vi "GRIMMcontrollerVI.vi"(8 "error in (no error)":errorcluster) -> (0 "error out":errorcluster)   [LabVIEW 2013]
doc: "Use this template to build a VI to use as a subVI."
uses:
  GRIMMstatusEnum.ctl
  GRIMMmeasurementEnum.ctl
  GRIMMErrorMessage.ctl
  GRIMMmeasurementCluster.ctl
  <vilib>/Instr/_visa.llb/VISA Configure Serial Port (Instr).vi
panel:
  in  "Save GRIMM file":bool
  in  "GRIMM File Path":path
  in  "error in (no error) 3":errorcluster
  out "XY Graph 2":cluster{dbl[], dbl[]}[](graph)
  out "Counts vs Time":waveform(dbl)[](graph)
  out "XY Graph":cluster{dbl[], dbl[]}[](graph)
  out "Error Messages":u16(ring) items=["New SELF-TEST: Fault Self-Test"=128, "No Memory Card"=64, "Check Nozzle: Whirls > 5%"=32, "No Operation: Battery Capacity = 0%"=16, "Please Recharge: Battery Capacity < 10%"=8, "Pump Current too High - Motor Current Imot > 100%"=4, "Flow-Error: Volume flow control out of control range"=3, "Check Filter Imot < 20% "=2, "Check Filter Imot > 60%"=1, "No Error :)"=0]
  out "Battery Power (%)":i32
  out "Power Supply Type":T1(ring)
  out "Pump Current (%)":i32
  out "Number of Particles":i32[](array[numeric])
  in  "error in (no error) 2":errorcluster
  in  "Set Interval Time Button":bool
  in  "Interval Time":T2(ring)
  out "read buffer":string
  in  "Stop GRIMM Measurement":bool
  in  "Start GRIMM Measurement":bool
  in  "stop":bool
  in  "GRIMM Com Port":refnum<visa-resource-name>="COM16"
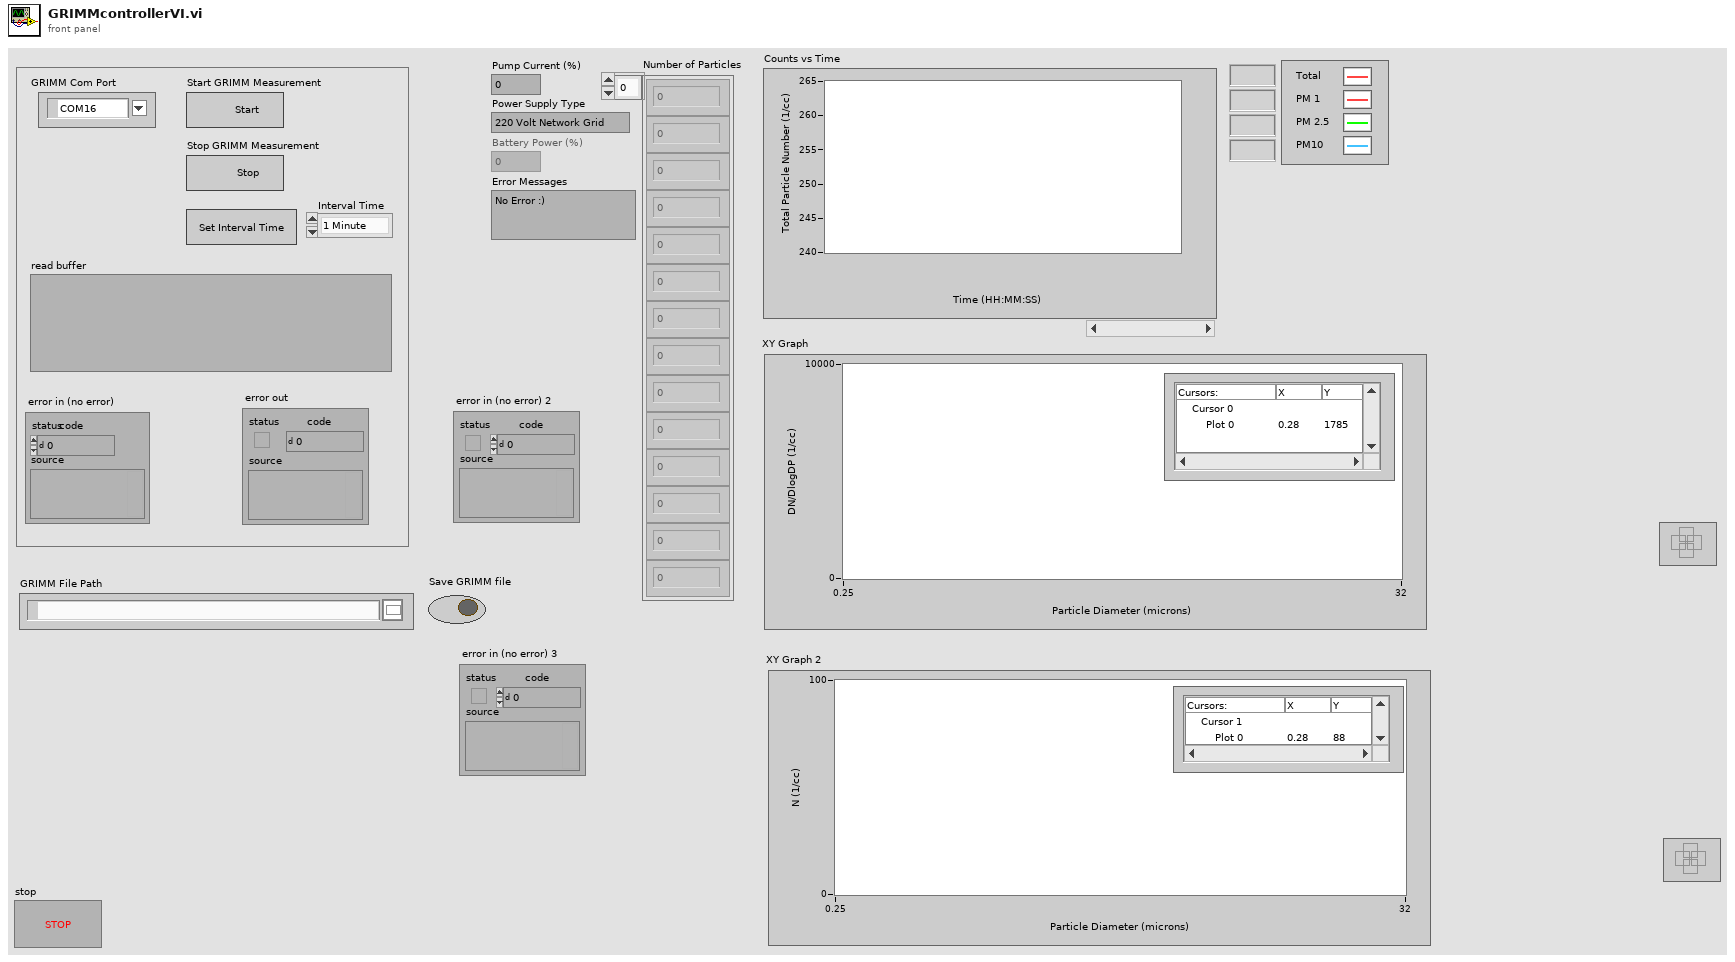
[diagram p1: front panel]
types:
  T1 = enum16{"220 Volt Network Grid", "Battery Powered"}
  T2 = enum16{"1 Minute", "5 Mintues", "10 Minutes", "15 Minutes", "30 Minutes", "60 Minutes", "6 Seconds", "3 Seconds", "2 Seconds", "1 Second"}
  T3 = typedef "GRIMMmeasurementEnum.ctl" = enum16{"Save Raw to file", "Get NvsDiameter", "Get DNDlogDPVsDiameter", "Get CountsVsTime", "Get Raw Data", "InsertMeasurement", "Init"}
  T4 = typedef "GRIMMstatusEnum.ctl" = enum16{"Get Pump Current", "Get Power Supply Type", "Get Battery Power", "Get Error message", "Get Instrument DateTime", "Insert Status Data", "Init"}
  T5 = typedef "GRIMMmeasurementCluster.ctl" = cluster{"Threshold Bin size":dbl[], "Measurement Data":i32[]}
  T6 = enum8{"Enabled", "Disabled", "Disabled and Grayed Out"}
  T7 = typedef "GRIMMErrorMessage.ctl" = u16
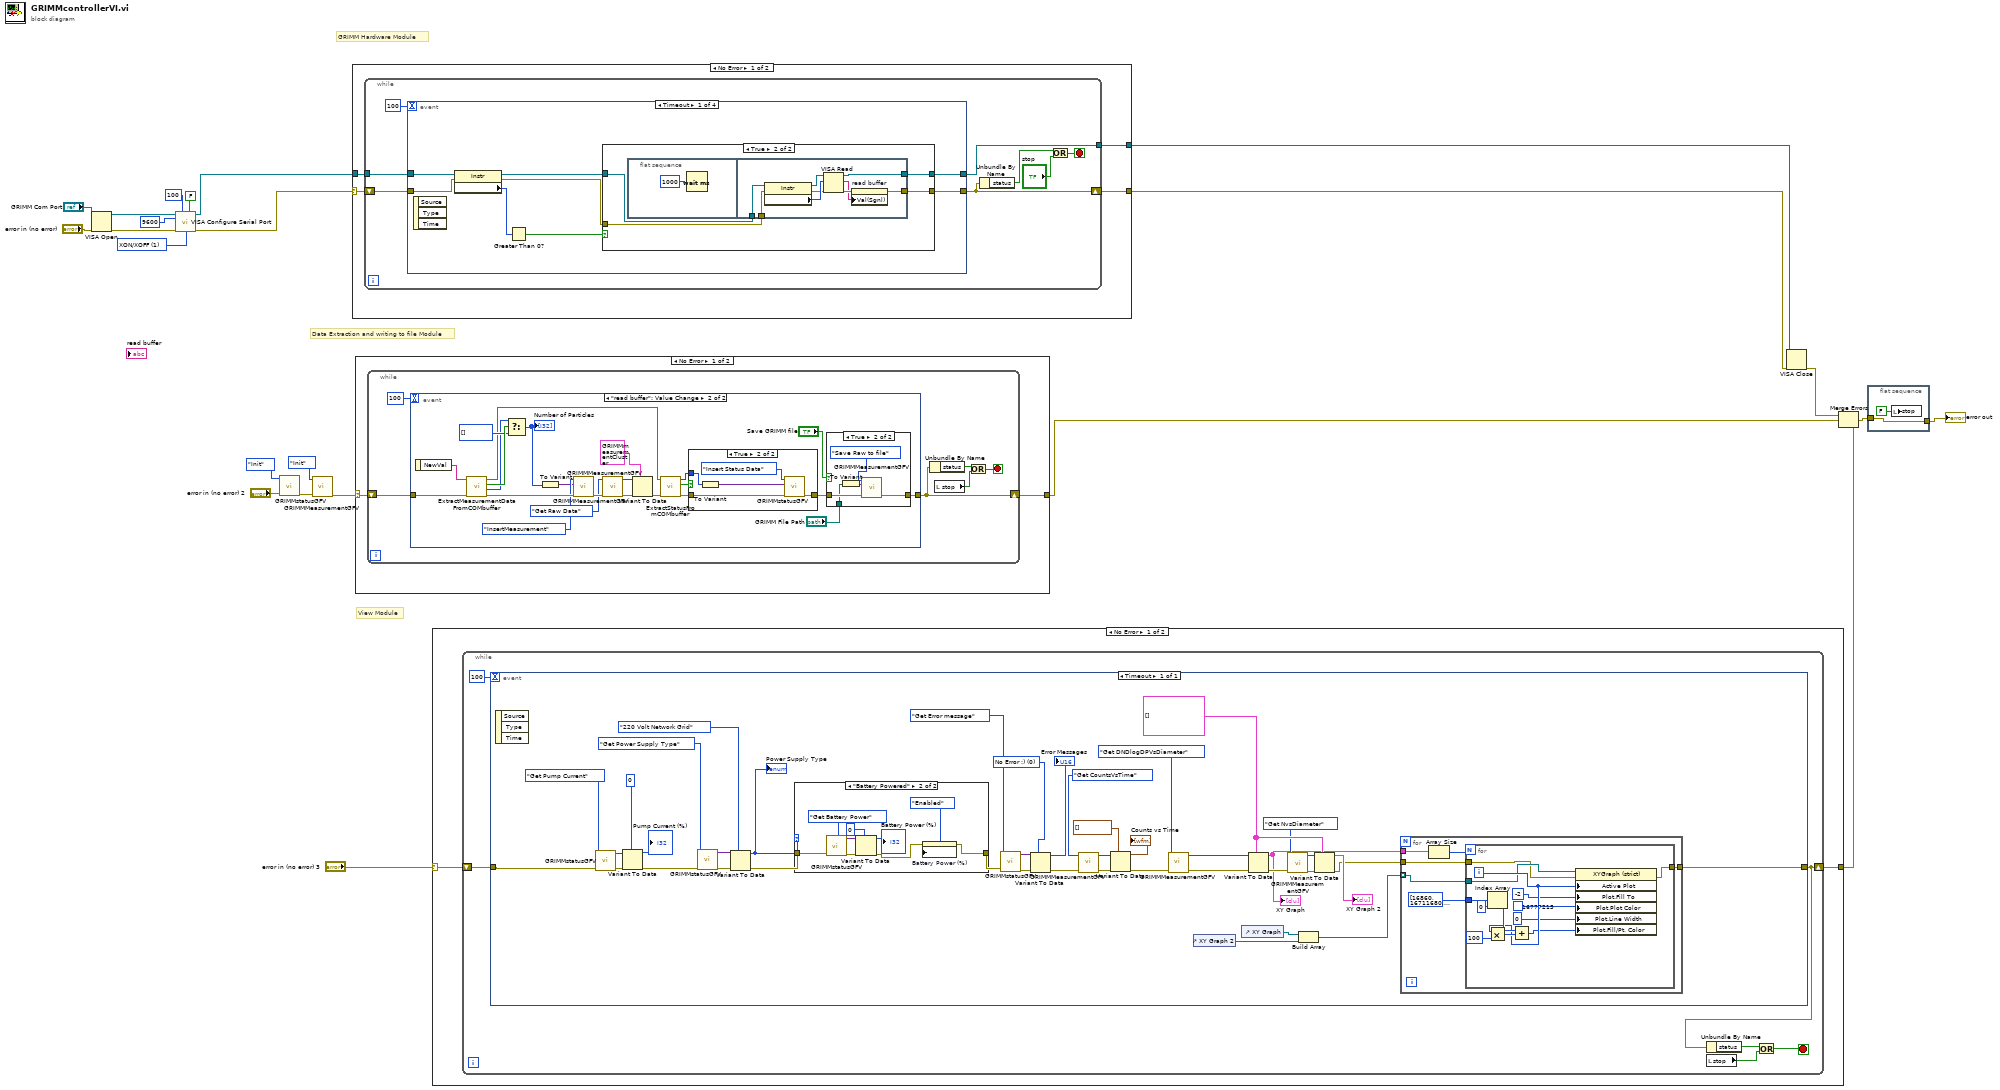
[diagram p0: block diagram]
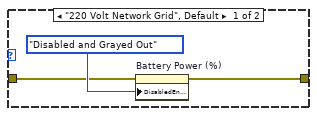
[diagram p2: hidden frame]
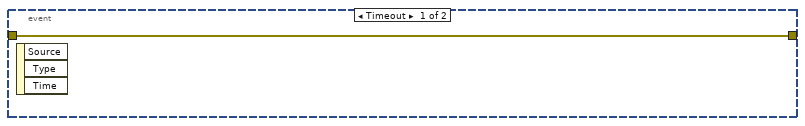
[diagram p4: hidden frame]
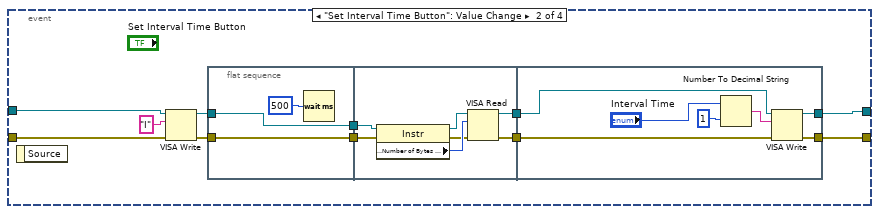
[diagram p9: hidden frame]
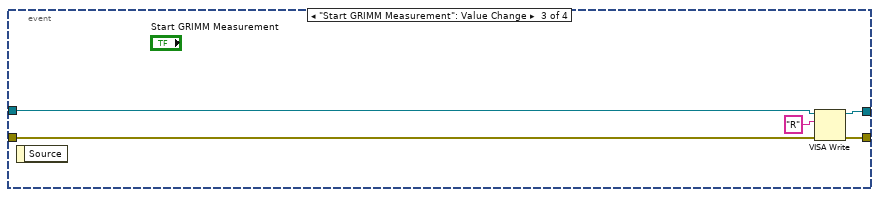
[diagram p10: hidden frame]
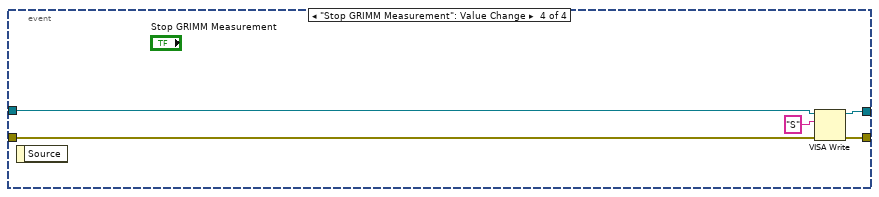
[diagram p11: hidden frame]
diagram:
  w16 = u16 1 items=["None", "XON/XOFF", "RTS/CTS", "XON/XOFF & RTS/CTS", "DTR/DSR", "XON/XOFF & DTR/DSR"] ("flow control (0:none)")
  # "View Module"
  # "Data Extraction and writing to file Module"
  # "GRIMM Hardware Module"
  n1 = VISA Open(error in (no error)="error in (no error)", VISA resource name="GRIMM Com Port") -> (VISA resource name=w23:refnum<visa-resource-name>, error out=w22:errorcluster)  [unwired: 3 in]
  n2 = call-poly "VISA Configure Serial Port"("VISA resource name"=w23, "timeout (10sec)"=u32 100, "Enable Termination\nChar (T)"=FALSE ("Enable Termination\nChar (T)"), "baud rate (9600)"=u32 9600, "error in (no error)"=w22, "flow control (0:none)"=w16) -> ("VISA resource name out"=w13:refnum<visa-resource-name>, "error out"=w15:errorcluster)  [unwired: 8 in]
  n3 = call "GRIMMstatusGFV.vi"("error in (no error)"="error in (no error) 2", "GrimmStatusEnum"=GRIMMstatusEnum."Init") -> ("error out"=w5:errorcluster)  [unwired: 8 in, 1 out]
  n4 = call "GRIMMMeasurementGFV.vi"("error in (no error)"=w5, "GRIMMMeasEnum"=GRIMMmeasurementEnum."Init") -> ("error out"=w3:errorcluster)  [unwired: 8 in, 1 out]
  n5 = case shown="No Error" w15 {
    selector: w15 -> [w26 w99]
    tunnel: [w25 w99] -> w14
    tunnel: w13 -> [w27 w98]
    tunnel: [w24 w98] -> w12
    frame No Error {
      n6 = while {
        tunnel: w27 -> [w34]
        tunnel: [w33] -> w24
        shift-right: [w32] -> w25
        shift-left: w26 -> [w35]
        stop <- w29 stop-if-true
        n7 = event shown="[0] Timeout" {
          selector: _ -> [_ _ _ _]
          dyn-events: _ -> [_ _ _ _]
          timeout: 100 -> [_ _ _ _]
          tunnel: w35 -> [w39 w70 w90 w95]
          tunnel: [w36 w62 w89 w94] -> w32
          tunnel: [w37 w61 w88 w93] -> w33
          tunnel: w34 -> [w43 w69 w91 w96]
          event Timeout {
            n8 = event-data() -> ()  [unwired: 1 in, 3 out]
            n9 = property class="Instr"(reference=w43, error in=w39) -> (reference out=w40:refnum<visa-resource-name>, error out=w38:errorcluster, "Serial Settings:Number of Bytes at Serial Port"=w41:u32)
            n10 = Greater Than 0?(x=w41) -> (x > 0?=w42:bool)
            n11 = case shown="True" w42 {
              tunnel: w40 -> [w44 w49]
              tunnel: w38 -> [w45 w48]
              tunnel: [w44 w47] -> w37
              tunnel: [w45 w46] -> w36
              frame False {
              }
              frame True {
                n12 = flat-sequence {
                  tunnel: w49 -> [w59]
                  tunnel: w48 -> [w56]
                  tunnel: [w54] -> w47
                  tunnel: [w52] -> w46
                  frame #0 {
                    n13 = Wait (ms)(milliseconds to wait=u32 1000) -> ()  [unwired: 1 out]
                  }
                  frame #1 {
                    n14 = property class="Instr"(reference=w59, error in=w56) -> (reference out=w58:refnum<visa-resource-name>, error out=w55:errorcluster, "Serial Settings:Number of Bytes at Serial Port"=w57:u32)
                    n15 = VISA Read(VISA resource name=w58, byte count=w57, error in (no error)=w55) -> (VISA resource name out=w54:refnum<visa-resource-name>, read buffer=w51:string, error out=w53:errorcluster)  [unwired: 1 out]
                    n16 = property on="read buffer" class="Str"(error in=w53, "Val(Sgnl)"=w51) -> (error out=w52:errorcluster)  [unwired: 1 in, 1 out]
                  }
                }
              }
            }
          }
          event "Set Interval Time Button": Value Change {
            n17 = event-data() -> ()  [unwired: 1 in, 1 out]
            n18 = VISA Write(VISA resource name=w69, write buffer="I" ("string"), error in (no error)=w70) -> (VISA resource name out=w67:refnum<visa-resource-name>, error out=w66:errorcluster)  [unwired: 1 out]
            n19 = flat-sequence {
              tunnel: w67 -> [w72]
              tunnel: w66 -> [w71]
              tunnel: [w72] -> w65
              tunnel: [w71] -> w60
              tunnel: w65 -> [w77]
              tunnel: [w76] -> w64
              tunnel: [w75] -> w63
              tunnel: w60 -> [w74]
              tunnel: w64 -> [w85]
              tunnel: w63 -> [w84]
              tunnel: [w83] -> w62
              tunnel: [w82] -> w61
              frame #0 {
                n20 = Wait (ms)(milliseconds to wait=u32 500) -> ()  [unwired: 1 out]
              }
              frame #1 {
                n21 = property class="Instr"(reference=w77, error in=w74) -> (reference out=w80:refnum<visa-resource-name>, error out=w78:errorcluster, "Serial Settings:Number of Bytes at Serial Port"=w79:u32)
                n22 = VISA Read(VISA resource name=w80, byte count=w79, error in (no error)=w78) -> (VISA resource name out=w76:refnum<visa-resource-name>, error out=w75:errorcluster)  [unwired: 2 out]
              }
              frame #2 {
                n23 = Number To Decimal String(number="Interval Time", width (-)=i16 1) -> (decimal integer string=w81:string)
                n24 = VISA Write(VISA resource name=w85, write buffer=w81, error in (no error)=w84) -> (VISA resource name out=w82:refnum<visa-resource-name>, error out=w83:errorcluster)  [unwired: 1 out]
              }
            }
          }
          event "Start GRIMM Measurement": Value Change {
            n25 = event-data() -> ()  [unwired: 1 in, 1 out]
            n26 = VISA Write(VISA resource name=w91, write buffer="R", error in (no error)=w90) -> (VISA resource name out=w88:refnum<visa-resource-name>, error out=w89:errorcluster)  [unwired: 1 out]
          }
          event "Stop GRIMM Measurement": Value Change {
            n27 = event-data() -> ()  [unwired: 1 in, 1 out]
            n28 = VISA Write(VISA resource name=w96, write buffer="S", error in (no error)=w95) -> (VISA resource name out=w93:refnum<visa-resource-name>, error out=w94:errorcluster)  [unwired: 1 out]
          }
        }
        n29 = Unbundle By Name(w32) -> ("status"=w31:bool)
        n30 = Or(x=w31, y="stop") -> (x .or. y?=w29:bool)
      }
    }
    frame Error {
    }
  }
  n31 = case shown="No Error" w3 {
    selector: w3 -> [w101 w144]
    tunnel: [w100 w144] -> w11
    frame No Error {
      n32 = while {
        shift-right: [w105] -> w100
        shift-left: w101 -> [w107]
        stop <- w102 stop-if-true
        n33 = event shown="[1] \"read buffer\": Value Change" {
          selector: _ -> [_ _]
          dyn-events: _ -> [_ _]
          timeout: 100 -> [_ _]
          tunnel: w107 -> [w108 w130]
          tunnel: [w108 w111] -> w105
          event Timeout {
            n34 = event-data() -> ()  [unwired: 1 in, 3 out]
          }
          event "read buffer": Value Change {
            n35 = event-data() -> ("NewVal"=w131:string)  [unwired: 1 in]
            n36 = call "ExtractMeasurementDataFromCOMbuffer.vi"("error in (no error)"=w130, "Input OPC data"=w131) -> ("error out"=w125:errorcluster, "Output Number of Particles per 100 CC"=w127:i32[], "Valid Data"=w129:bool, "Output OPC data"=w126:string)  [unwired: 6 in]
            n37 = Select(t=w127, s=w129, f=i32[] []) -> (s? t:f=w122:i32[])
            "Number of Particles" <- w122
            n38 = To Variant(anything=w122) -> (Variant=w123:variant)
            n39 = call "GRIMMMeasurementGFV.vi"("error in (no error)"=w125, "Variant in"=w123, "GRIMMMeasEnum"=GRIMMmeasurementEnum."InsertMeasurement") -> ("error out"=w121:errorcluster)  [unwired: 7 in, 1 out]
            n40 = call "GRIMMMeasurementGFV.vi"("error in (no error)"=w121, "GRIMMMeasEnum"=GRIMMmeasurementEnum."Get Raw Data") -> ("error out"=w115:errorcluster, "Variant out"=w117:variant)  [unwired: 8 in]
            n41 = Variant To Data(error in=w115, type=T5 {"Threshold Bin size"=[], "Measurement Data"=[0, 0, 0, 0, 0, 0, 0, 1, 1, 1, 1, 1, 1, 2, 2, 2, 2, 3, 4, 4, 5, 6, 8, 8, 10, 12, 15, 18, 20, 25, 30, 32]}, Variant=w117) -> (error out=w119:errorcluster)  [unwired: 1 out]
            n42 = call "ExtractStatusFromCOMbuffer.vi"("error in (no error)"=w119, "Input OPC data"=w126) -> ("error out"=w116:errorcluster, "Valid Data"=w114:bool, "GRIMM STATUS"=w113:i32[])  [unwired: 7 in]
            n43 = case shown="True" w114 {
              tunnel: w116 -> [w138 w143]
              tunnel: [w138 w142] -> w112
              tunnel: w113 -> [_ w139]
              frame False {
              }
              frame True {
                n44 = To Variant(anything=w139) -> (Variant=w140:variant)
                n45 = call "GRIMMstatusGFV.vi"("error in (no error)"=w143, "Variant in"=w140, "GrimmStatusEnum"=GRIMMstatusEnum."Insert Status Data") -> ("error out"=w142:errorcluster)  [unwired: 7 in, 1 out]
              }
            }
            n46 = case shown="True" "Save GRIMM file" {
              tunnel: w112 -> [w132 w137]
              tunnel: [w132 w136] -> w111
              tunnel: "GRIMM File Path" -> [_ w134]
              frame False {
              }
              frame True {
                n47 = To Variant(anything=w134) -> (Variant=w135:variant)
                n48 = call "GRIMMMeasurementGFV.vi"("error in (no error)"=w137, "Variant in"=w135, "GRIMMMeasEnum"=GRIMMmeasurementEnum."Save Raw to file") -> ("error out"=w136:errorcluster)  [unwired: 7 in, 1 out]
              }
            }
          }
        }
        n49 = Unbundle By Name(w105) -> ("status"=w104:bool)
        n50 = local read "stop"() -> (w103:bool)
        n51 = Or(x=w104, y=w103) -> (x .or. y?=w102:bool)
      }
    }
    frame Error {
    }
  }
  n52 = case shown="No Error" "error in (no error) 3" {
    selector: "error in (no error) 3" -> [w146 w225]
    tunnel: [w145 w225] -> w1
    frame No Error {
      n53 = while {
        shift-right: [w147] -> w145
        shift-left: w146 -> [w149]
        stop <- w150 stop-if-true
        n54 = event shown="[0] Timeout" {
          selector: _ -> [_]
          dyn-events: _ -> [_]
          timeout: 100 -> [_]
          tunnel: w149 -> [w155]
          tunnel: [w154] -> w147
          event Timeout {
            w189 = cluster{dbl[], dbl[]}[] []
            w171 = T7 0 items=["New SELF-TEST: Fault Self-Test"=128, "No Memory Card"=64, "Check Nozzle: Whirls > 5%"=32, "No Operation: Battery Capacity = 0%"=16, "Please Recharge: Battery Capacity < 10%"=8, "Pump Current too High - Motor Current Imot > 100%"=4, "Flow-Error: Volume flow control out of control range"=3, "Check Filter Imot < 20% "=2, "Check Filter Imot > 60%"=1, "No Error :)"=0] ("Error Messages")
            n55 = event-data() -> ()  [unwired: 1 in, 3 out]
            n56 = call "GRIMMstatusGFV.vi"("error in (no error)"=w155, "GrimmStatusEnum"=GRIMMstatusEnum."Get Pump Current") -> ("error out"=w157:errorcluster, "Variant out"=w158:variant)  [unwired: 8 in]
            n57 = Variant To Data(error in=w157, type=0 ("Pump Current %"), Variant=w158) -> (data=→"Pump Current (%)":i32, error out=w161:errorcluster)
            n58 = call "GRIMMstatusGFV.vi"("error in (no error)"=w161, "GrimmStatusEnum"=GRIMMstatusEnum."Get Power Supply Type") -> ("error out"=w163:errorcluster, "Variant out"=w164:variant)  [unwired: 8 in]
            n59 = Variant To Data(error in=w163, type=T1."220 Volt Network Grid" ("Power Supply"), Variant=w164) -> (data=w166:T1, error out=w167:errorcluster)
            "Power Supply Type" <- w166
            n60 = case shown="\"Battery Powered\"" w166 {
              tunnel: w167 -> [w214 w224]
              tunnel: [w213 w216] -> w168
              frame "220 Volt Network Grid", Default {
                n61 = property on="Battery Power (%)" class="DigNum (strict)"(error in=w214, "DisabledEnum"=T6."Disabled and Grayed Out" ("Disabled")) -> (error out=w213:errorcluster)  [unwired: 1 in, 1 out]
              }
              frame "Battery Powered" {
                n62 = call "GRIMMstatusGFV.vi"("error in (no error)"=w224, "GrimmStatusEnum"=GRIMMstatusEnum."Get Battery Power") -> ("error out"=w222:errorcluster, "Variant out"=w221:variant)  [unwired: 8 in]
                n63 = Variant To Data(error in=w222, type=0 ("Pump Current %"), Variant=w221) -> (data=→"Battery Power (%)":i32, error out=w218:errorcluster)
                n64 = property on="Battery Power (%)" class="DigNum (strict)"(error in=w218, "DisabledEnum"=T6."Enabled" ("Disabled")) -> (error out=w216:errorcluster)  [unwired: 1 in, 1 out]
              }
            }
            n65 = call "GRIMMstatusGFV.vi"("error in (no error)"=w168, "GrimmStatusEnum"=GRIMMstatusEnum."Get Error message") -> ("error out"=w170:errorcluster, "Variant out"=w173:variant)  [unwired: 8 in]
            n66 = Variant To Data(error in=w170, type=w171, Variant=w173) -> (data=→"Error Messages":T7, error out=w178:errorcluster)
            n67 = call "GRIMMMeasurementGFV.vi"("error in (no error)"=w178, "GRIMMMeasEnum"=GRIMMmeasurementEnum."Get CountsVsTime") -> ("error out"=w175:errorcluster, "Variant out"=w176:variant)  [unwired: 8 in]
            n68 = Variant To Data(error in=w175, type=waveform(dbl)[] [] ("appended array"), Variant=w176) -> (data=→"Counts vs Time":waveform(dbl)[], error out=w179:errorcluster)
            n69 = call "GRIMMMeasurementGFV.vi"("error in (no error)"=w179, "GRIMMMeasEnum"=GRIMMmeasurementEnum."Get DNDlogDPVsDiameter") -> ("error out"=w182:errorcluster, "Variant out"=w181:variant)  [unwired: 8 in]
            n70 = control-ref of="XY Graph 2"() -> (w192:refnum<vi>)
            n71 = control-ref of="XY Graph"() -> (w191:refnum<vi>)
            n72 = Variant To Data(error in=w182, type=w189, Variant=w181) -> (data=w183:cluster{dbl[], dbl[]}[], error out=w185:errorcluster)
            "XY Graph" <- w183
            n73 = call "GRIMMMeasurementGFV.vi"("error in (no error)"=w185, "GRIMMMeasEnum"=GRIMMmeasurementEnum."Get NvsDiameter") -> ("error out"=w187:errorcluster, "Variant out"=w188:variant)  [unwired: 8 in]
            n74 = Build Array(w191, w192) -> (w193:refnum<vi>[])
            n75 = Variant To Data(error in=w187, type=w189, Variant=w188) -> (data=→"XY Graph 2":cluster{dbl[], dbl[]}[], error out=w153:errorcluster)
            n76 = for {
              tunnel: [w198] -> w154
              tunnel: w183 -> [w197]
              tunnel: w193 -> [w195] mode=indexing
              tunnel: w153 -> [w194]
              n77 = Array Size(array=w197) -> (size(s)=w196:i32)
              n78 = for {
                N: w196 -> [_]
                tunnel: u32[] [16860, 16711680, 1175296, 16773632, 15679744, 16711925, 2818015, 4325415] -> [w212]
                tunnel: [w202] -> w198
                tunnel: w195 -> [w201]
                tunnel: w194 -> [w200]
                i -> [w207]
                n79 = Multiply(x=w207, y=100) -> (x*y=w209:i32)
                n80 = Index Array(array=w212, index=0) -> (element=w210:u32)
                n81 = Add(x=w210, y=w209) -> (x+y=w203:u32)
                n82 = property class="XYGraph (strict)"(reference=w201, error in=w200, "Active Plot"=w207, "Plot.Fill To"=i16 -2, "Plot.Plot Color"=u32 16777215, "Plot.Line Width"=u8 0, "Plot.Fill/Pt. Color"=w203) -> (error out=w202:errorcluster)  [unwired: 1 out]
              }
            }
          }
        }
        n83 = Unbundle By Name(w147) -> ("status"=w152:bool)
        n84 = local read "stop"() -> (w151:bool)
        n85 = Or(x=w152, y=w151) -> (x .or. y?=w150:bool)
      }
    }
    frame Error {
    }
  }
  n86 = VISA Close(VISA resource name=w12, error in (no error)=w14) -> (error out=w10:errorcluster)
  n87 = Merge Errors(w10, w11, w1) -> (w9:errorcluster)
  n88 = flat-sequence {
    tunnel: w9 -> [w226]
    tunnel: [w226] -> w8
    frame #0 {
      n89 = local write "stop"(FALSE ("stop")) -> ()
    }
  }
  "error out" <- w8
